vi "Create Evaluations.vi"(8 "error in (no error)":errorcluster, 11 "IEvaluation in":refnum<class "SpecAn_AMPM.lvclass">) -> (0 "error out":errorcluster, 2 "Evaluations Out":T1[](array[typedef]) {"Low Limit" format="%#_13g"; "SI Scaling" items=["femto"=-15, "pico"=-12, "nano"=-9, "micro"=-6, "milli"=-3, "percent"=-2, ""=0, "kilo"=3, "mega"=6, "giga"=9, "tera"=12]}, 3 "IEvaluation out":refnum<class "SpecAn_AMPM.lvclass">)   [LabVIEW 2018, in "SeqAuto Evaluations.lvlib" / "SpecAn_AMPM.lvclass"]
uses:
  SpecAn_AMPM.lvclass
  C:/Sequence Automation/Plugins/SeqAuto IEvaluation.lvlibp/SeqAuto IEvaluation.lvclass
  Plugins/TestStand API Tools (TSAT).lvlibp/Evaluation Actions/Includes/Controls/TSAT Evaluation.ctl
  Plugins/TestStand API Tools (TSAT).lvlibp/Evaluation Actions/Includes/Controls/TSAT Eval SI Unit Scaling.ctl
  Plugins/TestStand API Tools (TSAT).lvlibp/Evaluation Actions/Includes/Controls/TSAT Evaluation Type.ctl
  SpecAn_AMPM.lvclass/SpecAn_AMPM.ctl
  Read SA Pin.vi
  Plugins/SeqAuto IEvaluation.lvlibp/Read Measurement Name.vi
  Plugins/TestStand API Tools (TSAT).lvlibp/Evaluation Actions/TSAT Evaluation Actions.lvlib
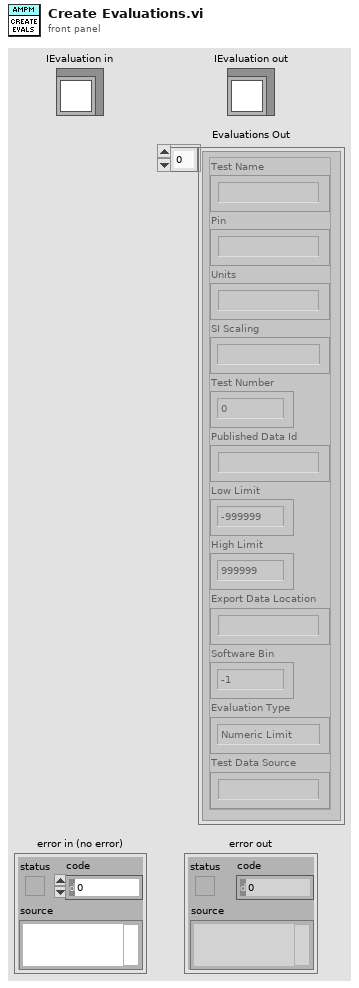
[diagram p1: front panel]
types:
  T1 = typedef "TestStand API Tools (TSAT).lvlibp/TSAT Evaluation Actions.lvlib/TSAT Evaluation.ctl" = cluster{"Test Name":string, "Pin":string, "Units":string, "SI Scaling":T2, "Test Number":i32, "Published Data Id":string, "Low Limit":dbl, "High Limit":dbl, "Export Data Location":string, "Software Bin":i64, "Evaluation Type":T3, "Test Data Source":string}
  T2 = typedef "TestStand API Tools (TSAT).lvlibp/TSAT Evaluation Actions.lvlib/TSAT Eval SI Unit Scaling.ctl" = i16
  T3 = typedef "TestStand API Tools (TSAT).lvlibp/TSAT Evaluation Actions.lvlib/TSAT Evaluation Type.ctl" = enum16{"Numeric Limit", "Pass/Fail", "None"}
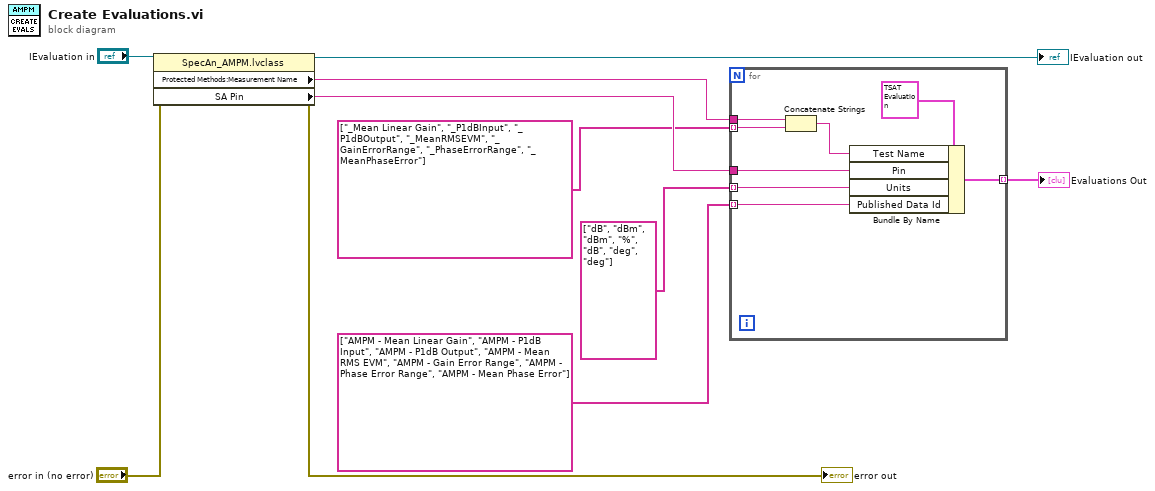
[diagram p0: block diagram]
diagram:
  n1 = property class="SpecAn_AMPM.lvclass"(reference="IEvaluation in", error in="error in (no error)") -> (reference out=→"IEvaluation out":refnum<class "SpecAn_AMPM.lvclass">, error out=→"error out":errorcluster, "Protected Methods:Measurement Name"=w10:string, "SA Pin"=w9:string)
  n2 = for {
    tunnel: [w17] -> w4 mode=indexing
    tunnel: w10 -> [w12]
    tunnel: w9 -> [w15]
    tunnel: string[] ["dB", "dBm", "dBm", "%", "dB", "deg", "deg"] -> [w14] mode=indexing
    tunnel: string[] ["AMPM - Mean Linear Gain", "AMPM - P1dB Input", "AMPM - P1dB Output", "AMPM - Mean RMS EVM", "AMPM - Gain Error Range", "AMPM - Phase Error Range", "AMPM - Mean Phase Error"] -> [w13] mode=indexing
    tunnel: string[] ["_Mean Linear Gain", "_P1dBInput", "_P1dBOutput", "_MeanRMSEVM", "_GainErrorRange", "_PhaseErrorRange", "_MeanPhaseError"] -> [w11] mode=indexing
    n3 = Concatenate Strings(w12, w11) -> (w16:string)
    n4 = Bundle By Name(cluster=T1 {"Test Name"="", "Pin"="", "Units"="", "SI Scaling"=0, "Test Number"=0, "Published Data Id"="", "Low Limit"=-999999.0, "High Limit"=999999.0, "Export Data Location"="", "Software Bin"=-1, "Evaluation Type"=enum."Numeric Limit", "Test Data Source"=""} ("Evaluation"), "Test Name"=w16, "Pin"=w15, "Units"=w14, "Published Data Id"=w13) -> (w17:T1)
  }
  "Evaluations Out" <- w4
